vi "Write time digit.vi"(8 "error in (no error)":errorcluster, 10 "Time":dbl, 11 "Abstract Display in":refnum<class "Abstract Display.lvclass">) -> (0 "error out":errorcluster, 3 "Abstract Display out":refnum<class "Abstract Display.lvclass">)   [LabVIEW 2012, in "Display Panel.lvlib" / "Abstract Display.lvclass"]
uses:
  Abstract Display.lvclass
  Abstract Display.lvclass/Abstract Display.ctl
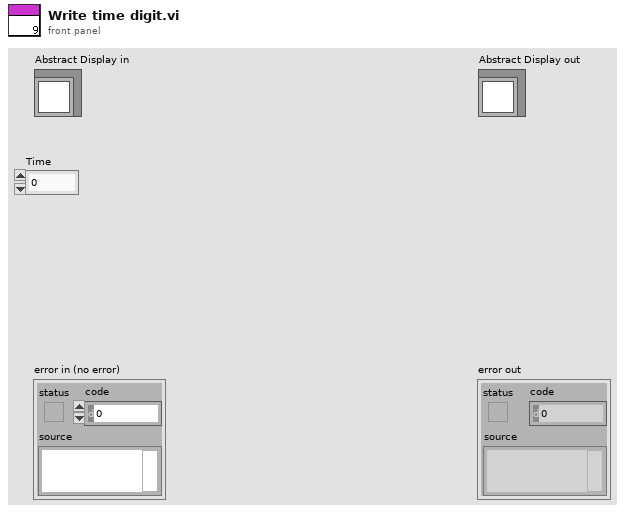
[diagram p1: front panel]
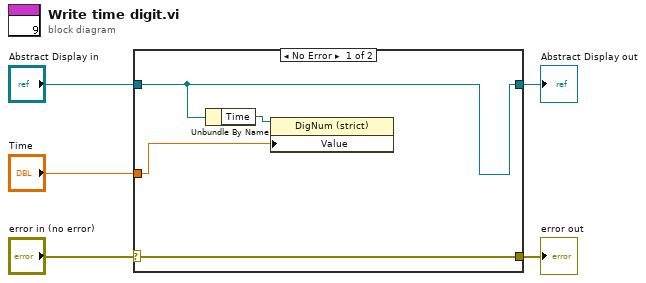
[diagram p0: block diagram]
diagram:
  n1 = case shown="No Error" "error in (no error)" {
    selector: "error in (no error)" -> [w9 w10]
    tunnel: [w9 w10] -> w4
    tunnel: [w8 w11] -> w2
    tunnel: "Abstract Display in" -> [w8 w11]
    tunnel: "Time" -> [w6 _]
    frame No Error {
      n2 = Unbundle By Name(w8) -> ("Time"=w7:refnum<vi>)
      n3 = property class="DigNum (strict)"(reference=w7, "Value"=w6) -> ()  [unwired: 1 in, 2 out]
    }
    frame Error {
    }
  }
  "error out" <- w4
  "Abstract Display out" <- w2
